vi "Get Abs Manual File Path.vi"(2 "error in (no error)":errorcluster, 3 "Application directory":path) -> (0 "error out":errorcluster, 1 "Manual file path":path)   [LabVIEW 2018, in "Tracker.lvlib"]
uses:
  Tracker.lvlib
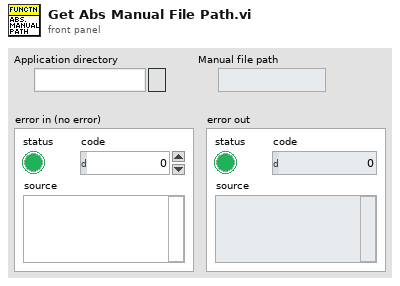
[diagram p1: front panel]
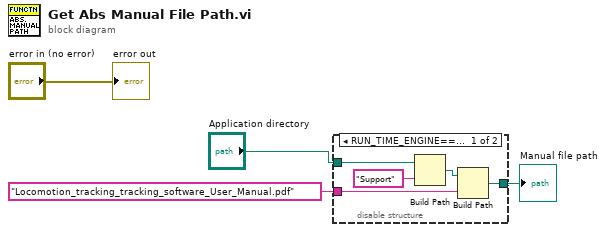
[diagram p0: block diagram]
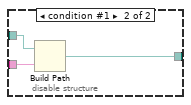
[diagram p2: hidden frame]
diagram:
  n1 = disable-structure shown="RUN_TIME_ENGINE==False" {
    disable-tunnel: "Application directory" -> [w5 w10]
    disable-tunnel: "Locomotion_tracking_tracking_software_User_Manual.pdf" ("name or relative path") -> [w7 w12]
    disable-tunnel: [w6 w11] -> w1
    frame condition #0 (active) {
      n2 = Build Path(base path=w5, name or relative path="Support") -> (appended path=w8:path)
      n3 = Build Path(base path=w8, name or relative path=w7) -> (appended path=w6:path)
    }
    frame condition #1 {
      n4 = Build Path(base path=w10, name or relative path=w12) -> (appended path=w11:path)
    }
  }
  "Manual file path" <- w1
  "error out" <- "error in (no error)"
